vi "Post-Install Custom Action.vi"(10 "Variant":variant) -> (0 "error out":errorcluster={"status"=TRUE, "code"=7, "source"="Invoke Node in GetTargetBuildSpecs.vi->NI_App_Builder_API.lvlib:Build (path).vi->Post-Install Custom Action.vi\n<APPEND>\nMethod Name: <b>Project:Open</b>"})   [LabVIEW 2017]
uses:
  <vilib>/AppBuilder/AB_API_Simple/NI_App_Builder_API.lvlib
  <vilib>/AppBuilder/AB_API_Simple/Build (path).vi
  <userlib>/NEVSTOP-Programming-Palette/Dialog & Interface/Fit VI window to Largest Dec_nevstop.vi
panel:
  in  "Tab Control":T1(tab)=enum."import registry patch"
  out "LabVIEW Version Selector lvproj Path":path
  in  "administrator privilege":bool
  in  "Normal Privilege":bool
  in  "introduction":string="Embed requesting administrator privilege menifest file to LabVIEW Version Selector application?\n\nIf Yes, LabVIEW launched by LabVIEW Version Selector will be run in administrator previlege everytime. \nYou can also rebuild with another option with the LabVIEW project if needed."
  in  "introduction 2":string="LabVIEW is now building the LabVIEW Version Selector...\n\n"
  in  "introduction 3":string="Import Registry Patch for Default Open application...\n\nIf you plan to import the registry manually, please double click the registry path file to add\nLabVIEW Version Selector to file open option list. "
  in  "Manually Later":bool
  in  "Import Now":bool
  in  "Finish":bool
  in  "introduction 4":string="Set LabVIEW Version Selector as first option as shown left. \n\nIf install.reg is not imported, you can select \"More apps\" to select LabVIEW Version Selector.exe in [LabVIEW]\\project\\_NEVSTOP\\LabVIEW-Version-Selector\\Build"
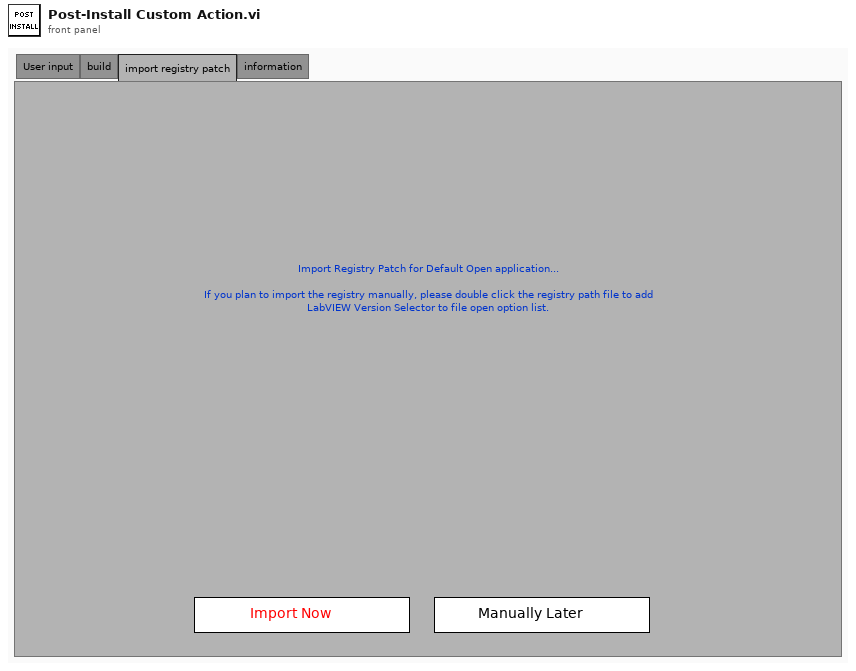
[diagram p1: front panel]
types:
  T1 = enum32{"User input", "build", "import registry patch", "information"}
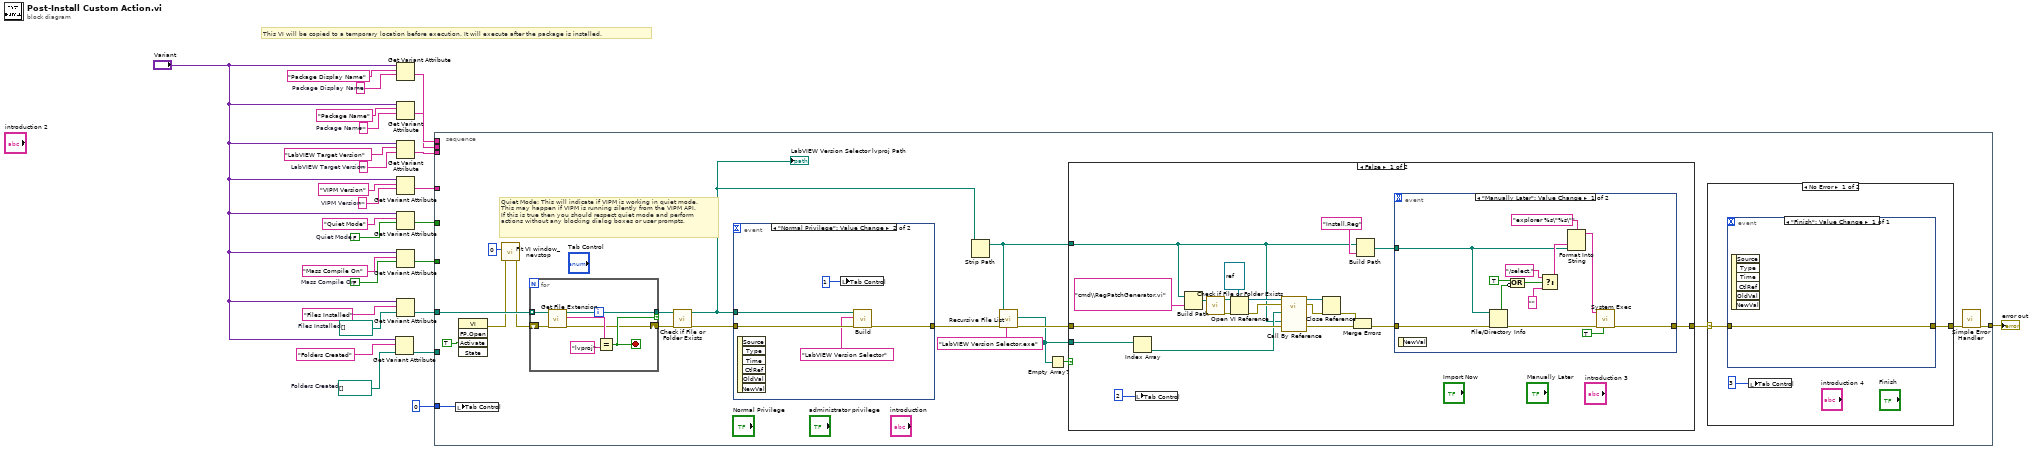
[diagram p0: block diagram]
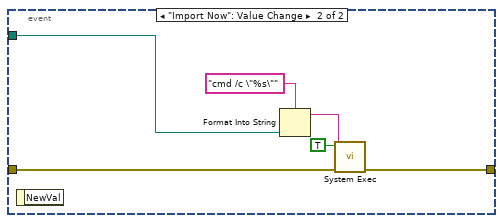
[diagram p3: hidden frame]
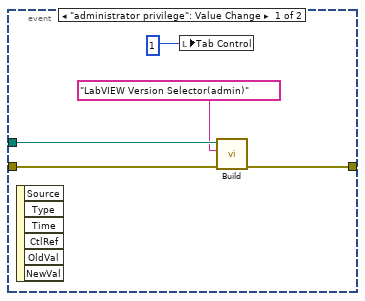
[diagram p5: hidden frame]
diagram:
  w3 = path[] []  # Folders Created
  w4 = path[] []  # Files Installed
  w10 = FALSE  # Mass Compile On
  w11 = ""  # Package Display Name
  w18 = FALSE  # Quiet Mode
  w21 = ""  # VIPM Version
  w23 = ""  # LabVIEW Target Version
  w25 = ""  # Package Name
  # "This VI will be copied to a temporary location before execution. It will execute after the package is installed."
  n1 = Get Variant Attribute(Variant="Variant", name="Folders Created", default value (empty Variant)=w3) -> (value=w8:path[])  [unwired: 1 in, 3 out]
  n2 = Get Variant Attribute(Variant="Variant", name="Package Display Name", default value (empty Variant)=w11) -> (value=w17:string)  [unwired: 1 in, 3 out]
  n3 = Get Variant Attribute(Variant="Variant", name="Package Name", default value (empty Variant)=w25) -> (value=w16:string)  [unwired: 1 in, 3 out]
  n4 = Get Variant Attribute(Variant="Variant", name="LabVIEW Target Version", default value (empty Variant)=w23) -> (value=w15:string)  [unwired: 1 in, 3 out]
  n5 = Get Variant Attribute(Variant="Variant", name="VIPM Version", default value (empty Variant)=w21) -> (value=w14:string)  [unwired: 1 in, 3 out]
  n6 = Get Variant Attribute(Variant="Variant", name="Quiet Mode", default value (empty Variant)=w18) -> (value=w13:bool)  [unwired: 1 in, 3 out]
  n7 = Get Variant Attribute(Variant="Variant", name="Mass Compile On", default value (empty Variant)=w10) -> (value=w12:bool)  [unwired: 1 in, 3 out]
  n8 = Get Variant Attribute(Variant="Variant", name="Files Installed", default value (empty Variant)=w4) -> (value=w7:path[])  [unwired: 1 in, 3 out]
  n9 = stacked-sequence {
    tunnel: w17 -> [_]
    tunnel: w16 -> [_]
    tunnel: w15 -> [_]
    tunnel: w14 -> [_]
    tunnel: w13 -> [_]
    tunnel: w12 -> [_]
    tunnel: w7 -> [w46]
    tunnel: w8 -> [_]
    tunnel: [w31] -> w2
    tunnel: 0 -> [w30]
    frame #0 {
      # "Quiet Mode: This will indicate if VIPM is working in quiet mode.\nThis may happen if VIPM is running silently from the VIPM API.\nIf this is true then you should respect quiet mode and perform\nactions without any blocking dialog boxes or user prompts."
      # "You can use the data extracted from the variant for whatever work you need to do."
      n10 = local write "Tab Control"(w30) -> ()
      n11 = invoke class="VI" method="FP.Open"("Activate"=TRUE ("Activate?")) -> (error out=w35:errorcluster)  [unwired: 4 in, 4 out]
      n12 = call-poly <userlib>:"Fit VI window_nevstop.vi"("error in (no error)"=w35, "border spacing (2 px)"=0) -> ("error out"=w33:errorcluster)  [unwired: 4 in, 1 out]
      n13 = for {
        tunnel: w46 -> [w108] mode=indexing
        tunnel: [w107] -> w45 if=w105
        shift-right: [w103] -> w44
        shift-left: w33 -> [w102]
        stop <- w105 stop-if-true
        n14 = call <vilib>:"Get File Extension.vi"("error in (no error)"=w102, "file"=w108) -> ("error out"=w103:errorcluster, "lowercase file extension"=w104:string, "dup file"=w107:path)  [unwired: 5 in, 2 out]
        n15 = Equal?(x=w104, y="lvproj") -> (x = y?=w105:bool)
      }
      n16 = call <vilib>:"Check if File or Folder Exists.vi"("error in (no error)"=w44, "path"=w45) -> ("error out"=w43:errorcluster, "dup path"=w42:path)  [unwired: 7 in, 1 out]
      "LabVIEW Version Selector lvproj Path" <- w42
      n17 = event shown="[1] \"Normal Privilege\": Value Change" {
        selector: _ -> [_ _]
        dyn-events: _ -> [_ _]
        timeout: _ -> [_ _]
        tunnel: w42 -> [w96 w101]
        tunnel: w43 -> [w95 w100]
        tunnel: [w94 w99] -> w40
        event "administrator privilege": Value Change {
          n18 = event-data() -> ()  [unwired: 1 in, 6 out]
          n19 = local write "Tab Control"(1) -> ()
          n20 = call-poly <vilib>:"Build.vi"("error in (no error)"=w95, "Name of build specification (if empty: build all)"="LabVIEW Version Selector(admin)", "Path to project"=w96) -> ("error out"=w94:errorcluster)  [unwired: 7 in, 1 out]
        }
        event "Normal Privilege": Value Change {
          n21 = event-data() -> ()  [unwired: 1 in, 6 out]
          n22 = local write "Tab Control"(1) -> ()
          n23 = call-poly <vilib>:"Build.vi"("error in (no error)"=w100, "Name of build specification (if empty: build all)"="LabVIEW Version Selector", "Path to project"=w101) -> ("error out"=w99:errorcluster)  [unwired: 7 in, 1 out]
        }
      }
      n24 = Strip Path(path=w42) -> (stripped path=w36:path)  [unwired: 1 out]
      n25 = call <vilib>:"Recursive File List.vi"("pattern"="LabVIEW Version Selector.exe", "error in (no error)"=w40, "Folder Path"=w36) -> ("error out"=w39:errorcluster, "All Files in Dir"=w38:path[])  [unwired: 4 in, 3 out]
      n26 = Empty Array?(array=w38) -> (empty?=w37:bool)
      n27 = case shown="False" w37 {
        tunnel: [w53 w91] -> w29
        tunnel: w39 -> [w60 w91]
        tunnel: w38 -> [w71 _]
        tunnel: w36 -> [w52 _]
        frame False {
          n28 = Index Array(array=w71) -> (element=w57:path)  [unwired: 1 in]
          n29 = local write "Tab Control"(2) -> ()
          n30 = Build Path(base path=w52, name or relative path="cmd\\RegPatchGenerator.vi") -> (appended path=w62:path)
          n31 = call <vilib>:"Check if File or Folder Exists.vi"("path"=w62) -> ("error out"=w69:errorcluster, "dup path"=w63:path)  [unwired: 8 in, 1 out]
          n32 = Open VI Reference(type specifier VI Refnum (for type only)=refnum<vi> refnum, vi path=w63, error in (no error)=w69) -> (vi reference=w65:refnum<vi>, error out=w66:errorcluster)  [unwired: 3 in]
          n33 = call-by-ref "?"(reference=w65, error in=w66, "error in"=w60, "reg patch file"=w52, "exe path"=w57) -> (reference out=w67:refnum<vi>, error out=w68:errorcluster, 0:"error out"=w59:errorcluster)  [unwired: 7 in, 1 out]
          n34 = Close Reference(reference=w67, error in (no error)=w68) -> (error out=w58:errorcluster)
          n35 = Merge Errors(w58, w59) -> (w54:errorcluster)
          n36 = Build Path(base path=w52, name or relative path="Install.Reg") -> (appended path=w55:path)
          n37 = event shown="[0] \"Manually Later\": Value Change" {
            selector: _ -> [_ _]
            dyn-events: _ -> [_ _]
            timeout: _ -> [_ _]
            tunnel: w55 -> [w75 w85]
            tunnel: w54 -> [w73 w87]
            tunnel: [w72 w86] -> w53
            event "Manually Later": Value Change {
              n38 = event-data() -> ()  [unwired: 1 in, 1 out]
              n39 = File/Directory Info(path=w75, error in=w73) -> (directory=w77:bool, error out=w78:errorcluster)  [unwired: 5 out]
              n40 = Compound Arithmetic op=OR(TRUE ("Select Directory? (F: Open Directory)"), invert w77) -> (w79:bool)
              n41 = Select(t="/select," ("format string"), s=w79, f="") -> (s? t:f=w80:string)
              n42 = Format Into String(format string="explorer %s\"%s\"", w80, w75) -> (resulting string=w76:string)  [unwired: 2 in, 1 out]
              n43 = call <vilib>:"System Exec.vi"("run minimized? (F)"=TRUE, "error in (no error)"=w78, "command line"=w76) -> ("error out"=w72:errorcluster)  [unwired: 5 in, 3 out]
            }
            event "Import Now": Value Change {
              n44 = event-data() -> ()  [unwired: 1 in, 1 out]
              n45 = Format Into String(format string="cmd /c \"%s\"", w85) -> (resulting string=w90:string)  [unwired: 2 in, 1 out]
              n46 = call <vilib>:"System Exec.vi"("run minimized? (F)"=TRUE, "error in (no error)"=w87, "command line"=w90) -> ("error out"=w86:errorcluster)  [unwired: 5 in, 3 out]
            }
          }
        }
        frame True {
        }
      }
      n47 = case shown="No Error" w29 {
        selector: w29 -> [w49 w51]
        tunnel: [w48 w51] -> w28
        frame No Error {
          n48 = event shown="[0] \"Finish\": Value Change" {
            selector: _ -> [_]
            dyn-events: _ -> [_]
            timeout: _ -> [_]
            tunnel: w49 -> [w50]
            tunnel: [w50] -> w48
            event "Finish": Value Change {
              n49 = event-data() -> ()  [unwired: 1 in, 6 out]
            }
          }
          n50 = local write "Tab Control"(3) -> ()
        }
        frame Error {
        }
      }
      n51 = call <vilib>:"Simple Error Handler.vi"("error in (no error)"=w28) -> ("error out"=w31:errorcluster)  [unwired: 4 in, 4 out]
    }
  }
  "error out" <- w2
